vi "Host_Streams_convertClusters.vi"(10 "Actuators in":T1, 11 "Data in":T2={"cRIO Data"={"Time (ms)"=0.0, "24V Battery (V)"=0.0, "LowV Current (A)"=0.0, "Fiducial Sensor (V)"=0.0, "PV Pressure (psig)"=0.0, "Flow Sensor (V)"=0.0, "Temp Fairing (F)"=0.0, "Temp Reservoir (F)"=0.0, "HallEffect Right (in)"=0.0, "HallEffect Left (in)"=0.0, "PT Tank (psig)"=0.0, "PT Clamp Right (psig)"=0.0, "PT Clamp Left (psig)"=0.0, "PT Brake (psig)"=0.0, "PT Cooling (psig)"=0.0, "Displacement (ft)"=0.0, "Velocity (ft/s)"=0.0}, "IMU Data"={"x acceleration (g)"=0.0, "Pressure (psia)"=0.0, "Temperature (F)"=0.0}, "BMS Data"={"Max Cell Voltage (V)"=0.0, "Max Cell ID"=0.0, "Min Cell Voltage (V)"=0.0, "Min Cell ID"=0.0, "State of Charge (%)"=0.0, "Average Voltage (V)"=0.0, "Voltage Delta (V)"=0.0, "Pack Current (A)"=0.0, "Pack Voltage (V)"=0.0, "Max Resistance (Ohm)"=0.0, "Min Resistance (Ohm)"=0.0, "Average Resistance (Ohm)"=0.0, "Delta Resistance (Ohm)"=0.0, "Highest Temperature(F)"=0.0, "BmsStatus"={"isFault"=FALSE, "isolationMonitoring"=FALSE}}, "Motor Data"={"Velo (RPM)"=0.0, "MotorTemp(F)"=0.0, "CtrlTemp(F)"=0.0, "DcLinkVolt(V)"=0.0, "ErrorCode"=0.0, "motorStatus"={"isReady"=FALSE, "isOn"=FALSE, "isOperEn"=FALSE, "isFault"=FALSE, "isVoltEn"=FALSE, "targetReached"=FALSE, "isWarning"=FALSE}, "isAlive"=FALSE, "motorControllerState"=1}} {"Motor Data"."motorControllerState" items=["unknown"=1, "boot-up"=0, "stopped"=4, "operational"=5, "pre-operational"=127, "connection lost"=128]}) -> (2 "Name array":string[](array[string]), 3 "Info array":string[](array[string]))   [LabVIEW 2018]
doc: "Converts the clusters containing all of the data and actuators into a single string array. \nAlso creates a string array to hold the names of all of the columns."
uses:
  Master/DAQ/Master_DataControl.ctl
  Master/DAQ/TypeDef_cRIOData.ctl
  Master/IMU/TypeDef_IMUData.ctl
  Master/CAN/TypeDef_BMSData.ctl
  Master/CAN/TypeDef_BMS_Status.ctl
  Master/CAN/MotorController/fixedMotorData.ctl
  Master/CAN/MotorController/MotorStatus.ctl
  Master/Control/TypeDef_DigitalOuts.ctl
  Libraries/TypeDef_CurrentState.ctl
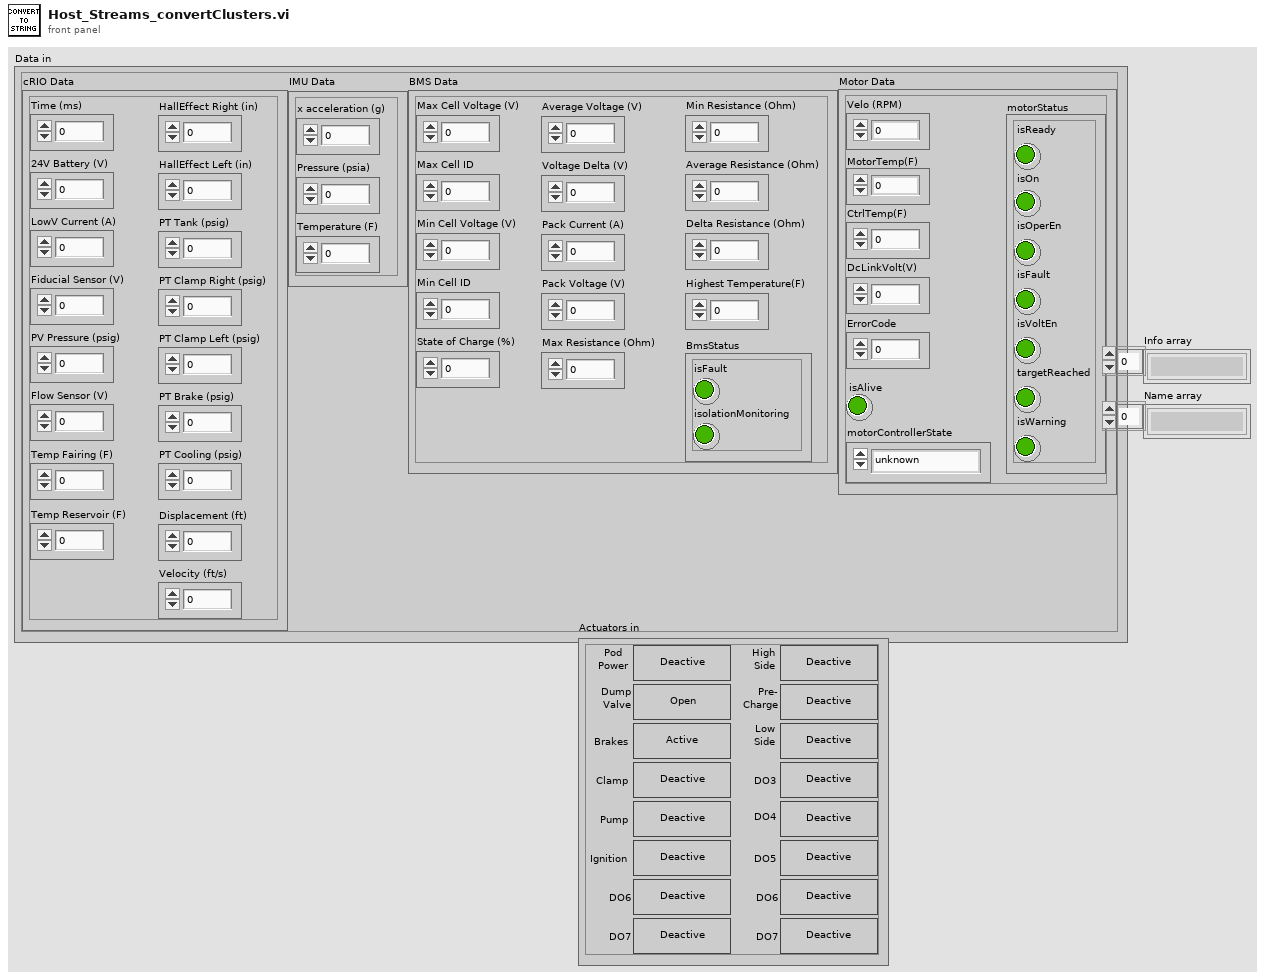
[diagram p1: front panel]
types:
  T1 = typedef "TypeDef_DigitalOuts.ctl" = cluster{"Pod Power":bool, "Dump Valve":bool, "Brakes":bool, "Clamp":bool, "Pump":bool, "Ignition":bool, "DO6":bool, "DO7":bool, "HighSide":bool, "Precharge":bool, "LowSide":bool, "DO3":bool, "DO4":bool, "DO5":bool, "DO62":bool, "DO72":bool}
  T2 = typedef "Master_DataControl.ctl" = cluster{"cRIO Data":T3, "IMU Data":T4, "BMS Data":T5, "Motor Data":T7}
  T3 = typedef "TypeDef_cRIOData.ctl" = cluster{"Time (ms)":dbl, "24V Battery (V)":dbl, "LowV Current (A)":dbl, "Fiducial Sensor (V)":dbl, "PV Pressure (psig)":dbl, "Flow Sensor (V)":dbl, "Temp Fairing (F)":dbl, "Temp Reservoir (F)":dbl, "HallEffect Right (in)":dbl, "HallEffect Left (in)":dbl, "PT Tank (psig)":dbl, "PT Clamp Right (psig)":dbl, "PT Clamp Left (psig)":dbl, "PT Brake (psig)":dbl, "PT Cooling (psig)":dbl, "Displacement (ft)":dbl, "Velocity (ft/s)":dbl}
  T4 = typedef "TypeDef_IMUData.ctl" = cluster{"x acceleration (g)":dbl, "Pressure (psia)":dbl, "Temperature (F)":dbl}
  T5 = typedef "TypeDef_BMSData.ctl" = cluster{"Max Cell Voltage (V)":dbl, "Max Cell ID":dbl, "Min Cell Voltage (V)":dbl, "Min Cell ID":dbl, "State of Charge (%)":dbl, "Average Voltage (V)":dbl, "Voltage Delta (V)":dbl, "Pack Current (A)":dbl, "Pack Voltage (V)":dbl, "Max Resistance (Ohm)":dbl, "Min Resistance (Ohm)":dbl, "Average Resistance (Ohm)":dbl, "Delta Resistance (Ohm)":dbl, "Highest Temperature(F)":dbl, "BmsStatus":T6}
  T6 = typedef "TypeDef_BMS_Status.ctl" = cluster{"isFault":bool, "isolationMonitoring":bool}
  T7 = typedef "fixedMotorData.ctl" = cluster{"Velo (RPM)":dbl, "MotorTemp(F)":dbl, "CtrlTemp(F)":dbl, "DcLinkVolt(V)":dbl, "ErrorCode":dbl, "motorStatus":T8, "isAlive":bool, "motorControllerState":u16}
  T8 = typedef "MotorStatus.ctl" = cluster{"isReady":bool, "isOn":bool, "isOperEn":bool, "isFault":bool, "isVoltEn":bool, "targetReached":bool, "isWarning":bool}
  T9 = typedef "TypeDef_CurrentState.ctl" = enum16{"Fault", "Idle", "Ready", "Pushing", "Coast", "Braking"}
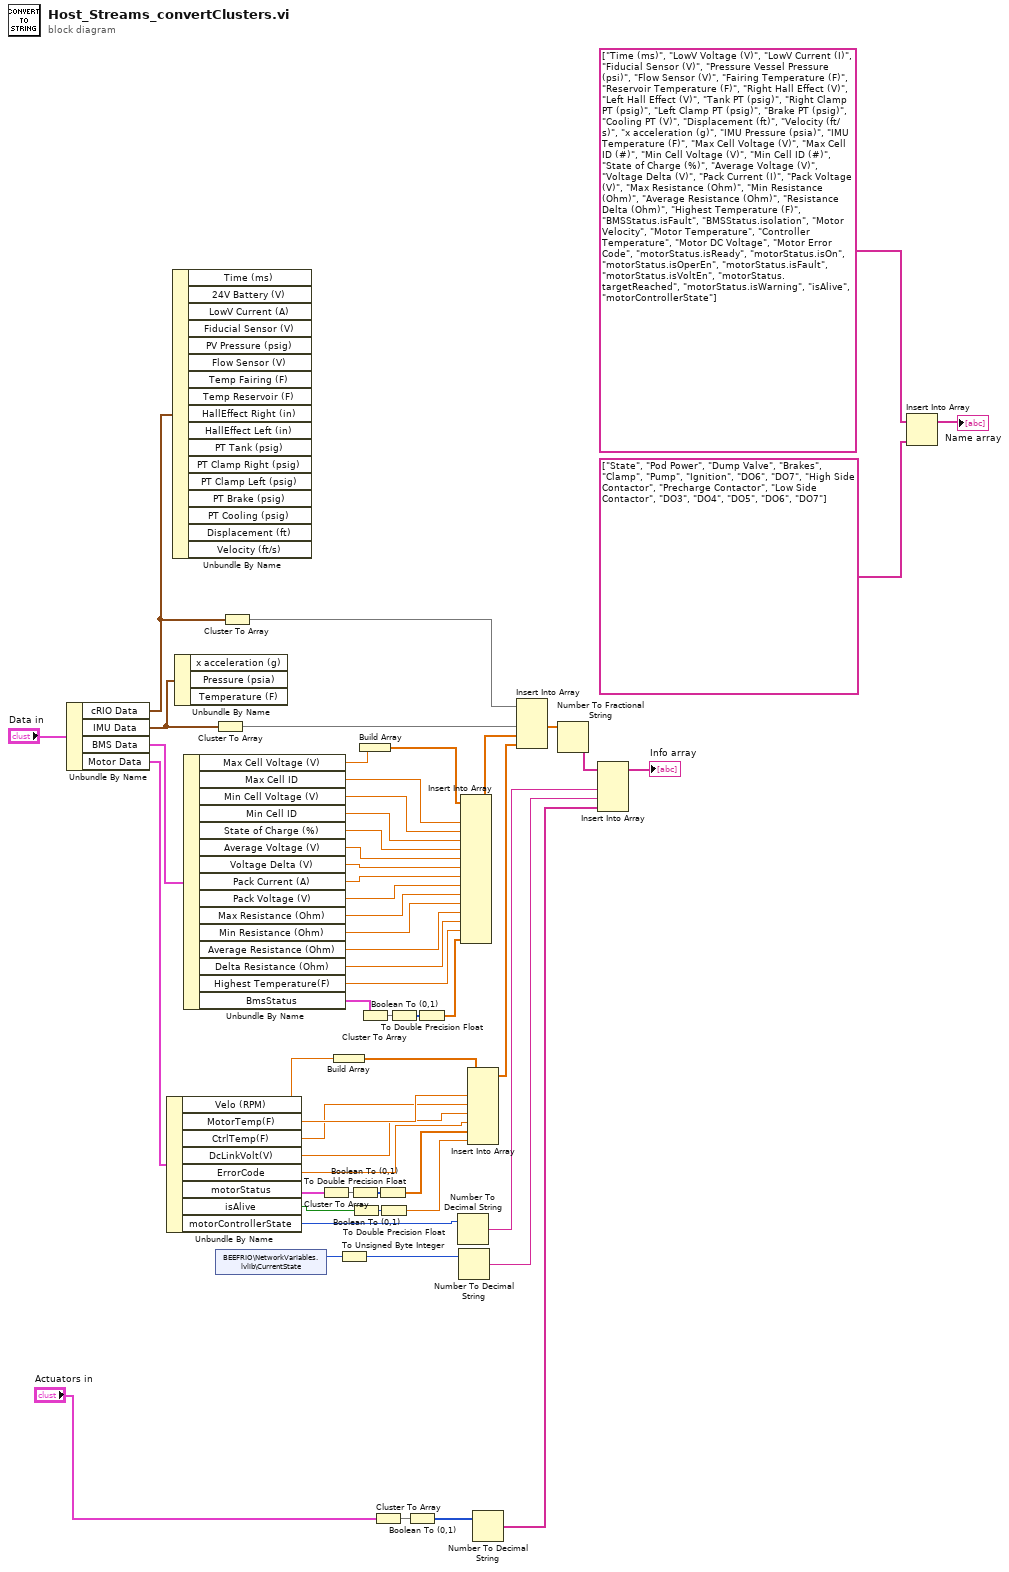
[diagram p0: block diagram]
diagram:
  n1 = Unbundle By Name("Data in") -> ("cRIO Data"=w55:T3, "IMU Data"=w54:T4, "BMS Data"=w40:T5, "Motor Data"=w39:T7)
  n2 = Unbundle By Name(w39) -> ("Velo (RPM)"=w35:dbl, "MotorTemp(F)"=w33:dbl, "CtrlTemp(F)"=w32:dbl, "DcLinkVolt(V)"=w31:dbl, "ErrorCode"=w30:dbl, "motorStatus"=w38:T8, "isAlive"=w27:bool, "motorControllerState"=w5:u16)
  n3 = Unbundle By Name(w55) -> ()  [unwired: 17 out]
  n4 = Unbundle By Name(w54) -> ()  [unwired: 3 out]
  n5 = Unbundle By Name(w40) -> ("Max Cell Voltage (V)"=w21:dbl, "Max Cell ID"=w19:dbl, "Min Cell Voltage (V)"=w18:dbl, "Min Cell ID"=w17:dbl, "State of Charge (%)"=w16:dbl, "Average Voltage (V)"=w15:dbl, "Voltage Delta (V)"=w14:dbl, "Pack Current (A)"=w13:dbl, "Pack Voltage (V)"=w12:dbl, "Max Resistance (Ohm)"=w11:dbl, "Min Resistance (Ohm)"=w10:dbl, "Average Resistance (Ohm)"=w9:dbl, "Delta Resistance (Ohm)"=w8:dbl, "Highest Temperature(F)"=w7:dbl, "BmsStatus"=w24:T6)
  n6 = Cluster To Array(cluster=w54) -> (array=w52:dbl[])
  n7 = shared-variable "BEEFRIO\\NetworkVariables.lvlib\\CurrentState"() -> (w42:T9)  [unwired: 1 in, 1 out]
  n8 = Cluster To Array(cluster=w55) -> (array=w53:dbl[])
  n9 = Cluster To Array(cluster=w38) -> (array=w36:bool[])
  n10 = Build Array(w35) -> (w34:dbl[])
  n11 = To Unsigned Byte Integer(number=w42) -> (unsigned 8bit integer=w41:u8)
  n12 = Boolean To (0,1)(Boolean=w36) -> (0, 1=w37:i16[])
  n13 = Boolean To (0,1)(Boolean=w27) -> (0, 1=w28:i16)
  n14 = Build Array(w21) -> (w20:dbl[])
  n15 = Cluster To Array(cluster=w24) -> (array=w23:bool[])
  n16 = Cluster To Array(cluster="Actuators in") -> (array=w48:bool[])
  n17 = To Double Precision Float(number=w37) -> (double precision float=w29:dbl[])
  n18 = To Double Precision Float(number=w28) -> (double precision float=w26:dbl)
  n19 = Boolean To (0,1)(Boolean=w23) -> (0, 1=w22:i16[])
  n20 = Boolean To (0,1)(Boolean=w48) -> (0, 1=w1:i16[])
  n21 = To Double Precision Float(number=w22) -> (double precision float=w6:dbl[])
  n22 = Number To Decimal String(number=w5) -> (decimal integer string=w2:string)  [unwired: 1 in]
  n23 = Number To Decimal String(number=w41) -> (decimal integer string=w3:string)  [unwired: 1 in]
  n24 = Insert Into Array(array=w20, new element #1=w19, new element #2=w18, new element #3=w17, new element #4=w16, new element #5=w15, new element #6=w14, new element #7=w13, new element #8=w12, new element #9=w11, new element #10=w10, new element #11=w9, new element #12=w8, new element #13=w7, new element #14=w6) -> (w51:dbl[])  [unwired: 1 in]
  n25 = Insert Into Array(array=w34, new element #1=w33, new element #2=w32, new element #3=w31, new element #4=w30, new element #5=w29, new element #6=w26) -> (w25:dbl[])  [unwired: 1 in]
  n26 = Number To Decimal String(number=w1) -> (decimal integer string=w4:string[])  [unwired: 1 in]
  n27 = Insert Into Array(array=w53, new element #1=w52, new element #2=w51, new element #3=w25) -> (w49:dbl[])  [unwired: 1 in]
  n28 = Number To Fractional String(number=w49) -> (F-format string=w47:string[])  [unwired: 3 in]
  n29 = Insert Into Array(array=w47, new element #1=w2, new element #2=w3, new element #3=w4) -> (→"Info array":string[])  [unwired: 1 in]
  n30 = Insert Into Array(array=string[] ["Time (ms)", "LowV Voltage (V)", "LowV Current (I)", "Fiducial Sensor (V)", "Pressure Vessel Pressure (psi)", "Flow Sensor (V)", "Fairing Temperature (F)", "Reservoir Temperature (F)", "Right Hall Effect (V)", "Left Hall Effect (V)", "Tank PT (psig)", "Right Clamp PT (psig)", "Left Clamp PT (psig)", "Brake PT (psig)", "Cooling PT (V)", "Displacement (ft)", "Velocity (ft/s)", "x acceleration (g)", "IMU Pressure (psia)", "IMU Temperature (F)", "Max Cell Voltage (V)", "Max Cell ID (#)", "Min Cell Voltage (V)", "Min Cell ID (#)", "State of Charge (%)", "Average Voltage (V)", "Voltage Delta (V)", "Pack Current (I)", "Pack Voltage (V)", "Max Resistance (Ohm)", "Min Resistance (Ohm)", "Average Resistance (Ohm)", "Resistance Delta (Ohm)", "Highest Temperature (F)", "BMSStatus.isFault", "BMSStatus.isolation", "Motor Velocity", "Motor Temperature", "Controller Temperature", "Motor DC Voltage", "Motor Error Code", "motorStatus.isReady", "motorStatus.isOn", "motorStatus.isOperEn", "motorStatus.isFault", "motorStatus.isVoltEn", "motorStatus.targetReached", "motorStatus.isWarning", "isAlive", "motorControllerState"], new element=string[] ["State", "Pod Power", "Dump Valve", "Brakes", "Clamp", "Pump", "Ignition", "DO6", "DO7", "High Side Contactor", "Precharge Contactor", "Low Side Contactor", "DO3", "DO4", "DO5", "DO6", "DO7"]) -> (→"Name array":string[])  [unwired: 1 in]
